vi "Read Epsilon.vi"(8 "error in (no error)":errorcluster, 11 "HG Observer in":refnum<class "HG Observer.lvclass">) -> (0 "error out":errorcluster, 2 "Epsilon":dbl, 3 "HG Observer out":refnum<class "HG Observer.lvclass">)   [LabVIEW 2014, in "Observer Library.lvlib" / "HG Observer.lvclass"]
uses:
  HG Observer.lvclass
  HG Observer.lvclass/HG Observer.ctl
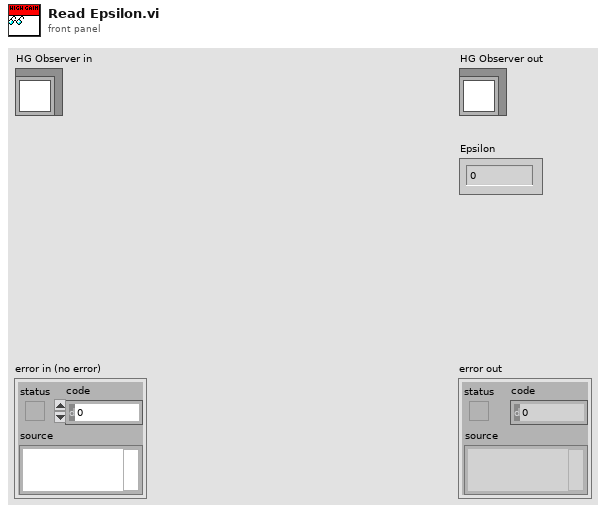
[diagram p1: front panel]
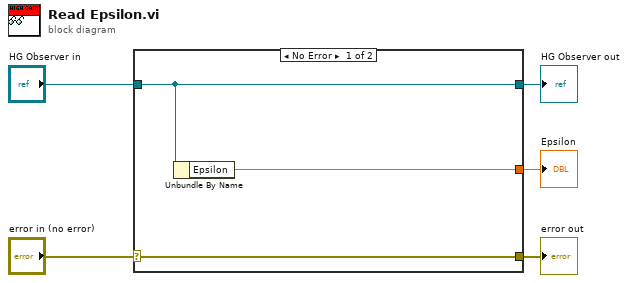
[diagram p0: block diagram]
diagram:
  n1 = case shown="No Error" "error in (no error)" {
    selector: "error in (no error)" -> [w8 w9]
    tunnel: [w8 w9] -> w4
    tunnel: [w7 w10] -> w2
    tunnel: "HG Observer in" -> [w7 w10]
    tunnel: [w6 _] -> w1
    frame No Error {
      n2 = Unbundle By Name(w7) -> ("Epsilon"=w6:dbl)
    }
    frame Error {
    }
  }
  "error out" <- w4
  "HG Observer out" <- w2
  "Epsilon" <- w1
